vi "[FPGA] DeltaSig Main V5.vi"() -> ()   [LabVIEW 2015]
doc: "This VI provides a template for customizing a waveform acquisition using delta-sigma based NI C Series analog input smodules."
uses:
  <vilib>/LabVIEW Targets/FPGA/cRIO/shared/nicrio_ModuleControls/nicrio_cRIO-9234_ConfigModeRing.ctl
  <vilib>/rvi/Emulation/niFpgaGetClockAttributes.vi
  <vilib>/rvi/Emulation/niFpgaSctlEmulationGetInTimedLoop.vi
  <vilib>/rvi/Emulation/niFpgaEmulationReportErrorSimple.vi
  <vilib>/LabVIEW Targets/FPGA/cRIO/shared/nicrio_DsaDataRateApi/_nicrio_9234GetDataRate131.vi
  <vilib>/rvi/Emulation/niFpgaProcessEmulError.vi
  <vilib>/rvi/eio/common/nirviEmuTemplatePropertySet_errors.vi
  <vilib>/rvi/eio/common/nirviEmuTemplateMethod_errors.vi
  <vilib>/rvi/interface/RandomDataEmulation/niFpgaRandomDataHandleErrors.vi
  <vilib>/rvi/Emulation/niFpgaCriticalErrorInLSC.vi
  <vilib>/eio/EIOPropertyNode/EIOPropertyNode.xnode
  <vilib>/LabVIEW Targets/FPGA/cRIO/shared/nicrio_ModuleControls/nicrio_cRIO-9234_DataRatesRing2.ctl
  <vilib>/eio/EIONode/EIONode.xnode
  <vilib>/rvi/DataTransferAndStorage/Container/XNode/niFpgaContainer.xnode
  <vilib>/rvi/interface/RandomDataEmulation/nirviRandomDataFpgaReadWriteTemplate.vi
  <vilib>/rvi/eio/common/nirviEmuTemplatePropertyGet_errors.vi
  <vilib>/rvi/eio/common/nirviEmuTemplatePropertyGet_noerrors.vi
  <vilib>/rvi/eio/common/nirviEmuTemplatePropertySet_noerrors.vi
panel:
  in  "Array Input Config":T1[](array[typedef])=[0, 0, 0, 0, 0, 0, 0, 0, 0, 0, 0, 0, 0, 0, 0, 0, 0, 0, 0, 0, 0, 0, 0, 0] items=["AC Coupled", "DC Coupled", "IEPE AC Coupled"]
  out "oclk freq":u32
  out "oclk div":u32
  out "oclk mult":u32
  in  "data rate (S/s)":u32
  in  "Chan Scale Array":sgl[](array[numeric])=[0.0, 0.0, 0.0, 0.0, 0.0, 0.0, 0.0, 0.0, 0.0, 0.0, 0.0, 0.0, 0.0, 0.0, 0.0, 0.0, 0.0, 0.0, 0.0, 0.0, 0.0, 0.0, 0.0, 0.0, 0.0, 0.0, 0.0, 0.0, 0.0, 0.0, 0.0, 0.0, 0.0, 0.0, 0.0, 0.0, 0.0, 0.0, 0.0, 0.0]
  out "Chan Count":bool
  out "Acq Loop Ticks":u32
  out "FPGA Error":errorcluster
  out "Module Underflow":bool
  out "Finished":bool
  in  "Number of Channels":i32=24
  in  "Samps per Chan [Finite]":i32=5120
  out "First Read":bool
  in  "Acquisition Type":enum16{"Finite Samples", "Continuous Samples"}(ring)
  out "DMA FIFO Full":bool
  in  "stop":bool
  # "Array size fixed at 40\nelements but may be \nexpanded if needed"
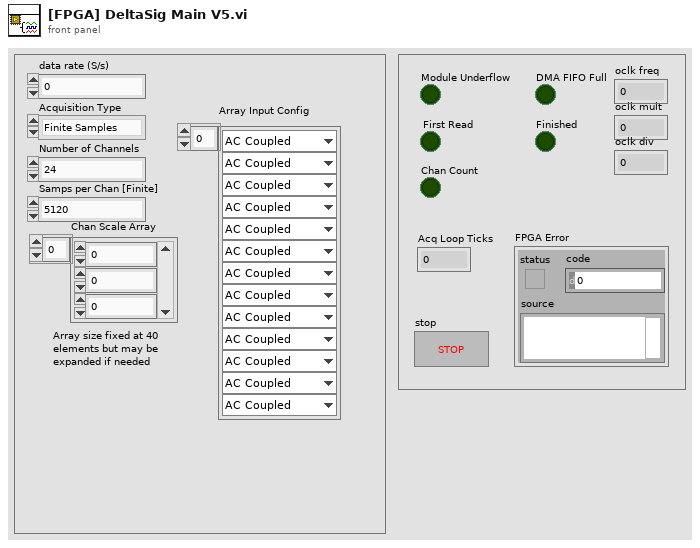
[diagram p1: front panel]
types:
  T1 = typedef "nicrio_cRIO-9234_ConfigModeRing.ctl" = u8
  T2 = typedef "nicrio_cRIO-9234_DataRatesRing2.ctl" = u8
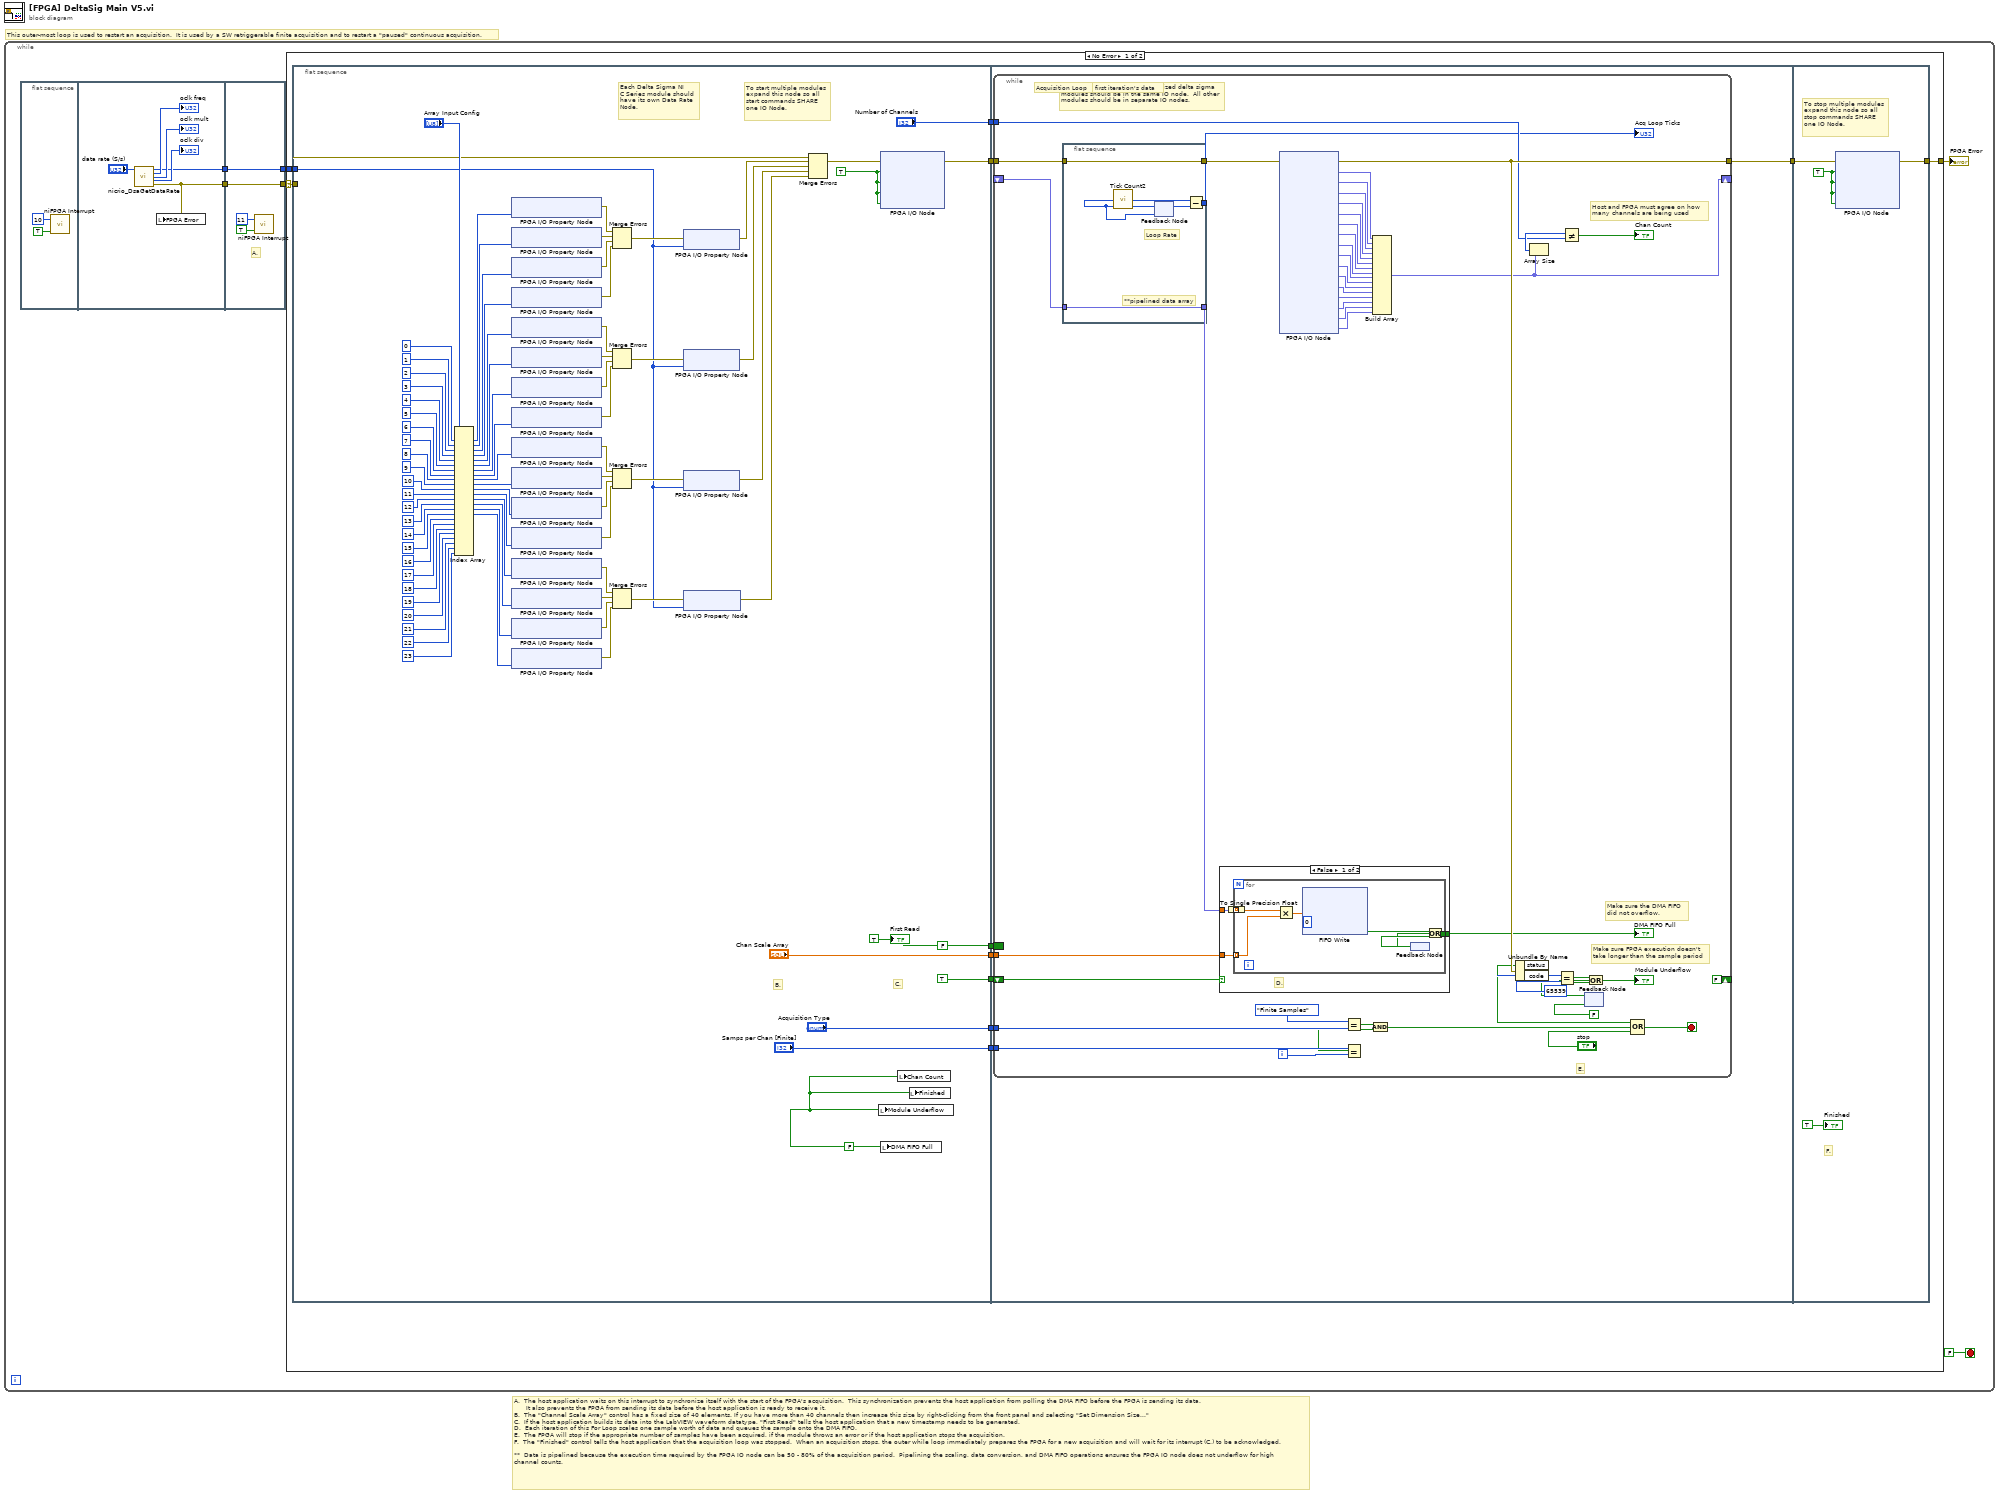
[diagram p0: block diagram]
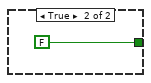
[diagram p2: hidden frame]
diagram:
  # "A.  The host application waits on this interrupt to synchronize itself with the start of the FPGA's acquisition.  This synchronization prevents the host application from polling the DMA FIFO before the FPGA is sending its data.\n      It also prevents the FPGA from sending its data before the host application is ready to receive it.\nB.  The \"Channel Scale Array\" control has a fixed size of 40 elements. If you have more than 40 channels then increase this size by right-clicking from the front panel and selecting \"Set Dimension Size...\"\nC.  If the host application builds its data into the LabVIEW waveform datatype, \"First Read\" tells the host application that a new timestamp needs to be generated.\nD.  Each iteration of this For Loop scales one sample worth of data and queues the sample onto the DMA FIFO.  \nE.  The FPGA will stop if the appropriate number of samples have been acquired, if the module throws an error or if the host application stops the acquisition.  \nF.  The \"Finished\" control tells the host application that the acquisition loop was stopped.  When an acquisition stops, the outer while loop immediately prepares the FPGA for a new acquisition and will wait for its interrupt (C.) to be acknowledged.\n\n**  Data is pipelined because the execution time required by the FPGA IO node can be 50 - 80% of the acquisition period.  Pipelining the scaling, data conversion, and DMA FIFO operations ensures the FPGA IO node does not underflow for high\nchannel counts."
  # "This outer-most loop is used to restart an acquisition.  It is used by a SW retriggerable finite acquisition and to restart a \"paused\" continuous acquisition."
  n1 = while {
    stop <- FALSE stop-if-true
    n2 = flat-sequence {
      tunnel: [w10] -> w2
      tunnel: [w11] -> w1
      tunnel: [w18] -> w3
      tunnel: [w15] -> w4
      tunnel: w2 -> [w15]
      tunnel: w1 -> [w18]
      frame #0 {
        n3 = call <vilib>:"niFPGA Interrupt.vi"("Wait Until Cleared (F)"=TRUE ("Wait Until Cleared"), "IRQ Number (0)"=u8 10 ("IRQ Number")) -> ()  [unwired: 1 in]
      }
      frame #1 {
        n4 = call-poly <vilib>:"nicrio_DsaGetDataRate.vi"("data rate (S/s)"="data rate (S/s)") -> ("data rate"=w11:T2, "oclk freq"=→"oclk freq":u32, "oclk mult"=→"oclk mult":u32, "oclk div"=→"oclk div":u32, "error out"=w10:errorcluster)  [unwired: 10 in]
        n5 = local write "FPGA Error"(w10) -> ()
      }
      frame #2 {
        # "A."
        n6 = call <vilib>:"niFPGA Interrupt.vi"("Wait Until Cleared (F)"=TRUE ("Wait Until Cleared"), "IRQ Number (0)"=u8 11 ("IRQ Number")) -> ()  [unwired: 1 in]
      }
    }
    n7 = case shown="No Error" w4 {
      selector: w4 -> [w19 w183]
      tunnel: [w21 w183] -> w5
      tunnel: w3 -> [w20 _]
      frame No Error {
        n8 = flat-sequence {
          tunnel: [w107] -> w29
          tunnel: ["Chan Scale Array"] -> w28
          tunnel: ["Acquisition Type"] -> w27
          tunnel: ["Samps per Chan [Finite]"] -> w26
          tunnel: ["Number of Channels"] -> w25
          tunnel: [TRUE ("t")] -> w24
          tunnel: [FALSE] -> w23
          tunnel: w20 -> [w30]
          tunnel: w19 -> [w79]
          tunnel: w29 -> [w114]
          tunnel: w28 -> [w113]
          tunnel: w27 -> [w111]
          tunnel: w26 -> [w110]
          tunnel: w25 -> [w115]
          tunnel: w24 -> [w112]
          tunnel: [w109] -> w22
          tunnel: w23 -> [w108]
          tunnel: w22 -> [w181]
          tunnel: [w180] -> w21
          frame #0 {
            w105 = FALSE ("Module Underflow")
            w31 = TRUE ("Mod1/Start")
            # "To start multiple modules\nexpand this node so all\nstart commands SHARE\none IO Node."
            # "C."
            # "B."
            # "Each Delta Sigma NI \nC Series module should \nhave its own Data Rate \nNode."
            n9 = Index Array(array="Array Input Config", index #1=0 ("index"), index #2=1 ("index"), index #3=2 ("index"), index #4=3 ("index"), index #5=4 ("index"), index #6=5 ("index"), index #7=6 ("index"), index #8=7 ("index"), index #9=8 ("index"), index #10=9 ("index"), index #11=10 ("index"), index #12=11 ("index"), index #13=12 ("index"), index #14=13 ("index"), index #15=14 ("index"), index #16=15 ("index"), index #17=16 ("index"), index #18=17 ("index"), index #19=18 ("index"), index #20=19 ("index"), index #21=20 ("index"), index #22=21 ("index"), index #23=22 ("index"), index #24=23 ("index")) -> (element #1=w97:T1, element #2=w96:T1, element #3=w95:T1, element #4=w94:T1, element #5=w75:T1, element #6=w74:T1, element #7=w73:T1, element #8=w72:T1, element #9=w59:T1, element #10=w58:T1, element #11=w57:T1, element #12=w56:T1, element #13=w55:T1, element #14=w53:T1, element #15=w52:T1, element #16=w51:T1)  [unwired: 8 out]
            n10 = xnode "FPGA I/O Property Node"("Input Configuration"=w97) -> ("error out"=w90:errorcluster)  [unwired: 2 in, 1 out]
            n11 = xnode "FPGA I/O Property Node"("Input Configuration"=w96) -> ("error out"=w89:errorcluster)  [unwired: 2 in, 1 out]
            n12 = xnode "FPGA I/O Property Node"("Input Configuration"=w95) -> ("error out"=w88:errorcluster)  [unwired: 2 in, 1 out]
            n13 = xnode "FPGA I/O Property Node"("Input Configuration"=w94) -> ("error out"=w87:errorcluster)  [unwired: 2 in, 1 out]
            n14 = xnode "FPGA I/O Property Node"("Input Configuration"=w75) -> ("error out"=w84:errorcluster)  [unwired: 2 in, 1 out]
            n15 = xnode "FPGA I/O Property Node"("Input Configuration"=w74) -> ("error out"=w83:errorcluster)  [unwired: 2 in, 1 out]
            n16 = xnode "FPGA I/O Property Node"("Input Configuration"=w73) -> ("error out"=w82:errorcluster)  [unwired: 2 in, 1 out]
            n17 = xnode "FPGA I/O Property Node"("Input Configuration"=w72) -> ("error out"=w81:errorcluster)  [unwired: 2 in, 1 out]
            n18 = xnode "FPGA I/O Property Node"("Input Configuration"=w59) -> ("error out"=w67:errorcluster)  [unwired: 2 in, 1 out]
            n19 = xnode "FPGA I/O Property Node"("Input Configuration"=w58) -> ("error out"=w66:errorcluster)  [unwired: 2 in, 1 out]
            n20 = xnode "FPGA I/O Property Node"("Input Configuration"=w57) -> ("error out"=w65:errorcluster)  [unwired: 2 in, 1 out]
            n21 = xnode "FPGA I/O Property Node"("Input Configuration"=w56) -> ("error out"=w64:errorcluster)  [unwired: 2 in, 1 out]
            n22 = xnode "FPGA I/O Property Node"("Input Configuration"=w55) -> ("error out"=w63:errorcluster)  [unwired: 2 in, 1 out]
            n23 = xnode "FPGA I/O Property Node"("Input Configuration"=w53) -> ("error out"=w62:errorcluster)  [unwired: 2 in, 1 out]
            n24 = xnode "FPGA I/O Property Node"("Input Configuration"=w52) -> ("error out"=w61:errorcluster)  [unwired: 2 in, 1 out]
            n25 = xnode "FPGA I/O Property Node"("Input Configuration"=w51) -> ("error out"=w60:errorcluster)  [unwired: 2 in, 1 out]
            n26 = Merge Errors(w90, w89, w88, w87) -> (w86:errorcluster)
            n27 = Merge Errors(w84, w83, w82, w81) -> (w80:errorcluster)
            n28 = Merge Errors(w67, w66, w65, w64) -> (w54:errorcluster)
            n29 = Merge Errors(w63, w62, w61, w60) -> (w34:errorcluster)
            n30 = xnode "FPGA I/O Property Node"("error in"=w86, "Data Rate"=w30) -> ("error out"=w77:errorcluster)  [unwired: 1 in, 1 out]
            n31 = xnode "FPGA I/O Property Node"("error in"=w80, "Data Rate"=w30) -> ("error out"=w76:errorcluster)  [unwired: 1 in, 1 out]
            n32 = xnode "FPGA I/O Property Node"("error in"=w54, "Data Rate"=w30) -> ("error out"=w33:errorcluster)  [unwired: 1 in, 1 out]
            n33 = xnode "FPGA I/O Property Node"("error in"=w34, "Data Rate"=w30) -> ("error out"=w32:errorcluster)  [unwired: 1 in, 1 out]
            n34 = Merge Errors(w79, w77, w76, w33, w32) -> (w78:errorcluster)
            n35 = local write "Module Underflow"(w105) -> ()
            n36 = xnode "FPGA I/O Node"("error in"=w78, "Mod1/Start"=w31, "Mod2/Start"=w31, "Mod3/Start"=w31, "Mod4/Start"=w31) -> ("error out"=w107:errorcluster)  [unwired: 4 in, 4 out]
            n37 = local write "DMA FIFO Full"(w105) -> ()
            n38 = local write "Chan Count"(w105) -> ()
            n39 = local write "Finished"(w105) -> ()
            "First Read" <- TRUE ("First Read")
          }
          frame #1 {
            n40 = while {
              tunnel: w114 -> [w151]
              tunnel: [w156] -> w109
              tunnel: w111 -> [w158]
              tunnel: w110 -> [w157]
              shift-right: [w131] -> _
              shift-left: _ -> [w144]
              tunnel: w115 -> [w153]
              tunnel: w113 -> [w145]
              shift-right: [FALSE ("t")] -> _
              shift-left: w112 -> [w143]
              border: w108 -> [_]
              i -> [w141]
              stop <- w128 stop-if-true
              # "Add channels here.  All synchronized delta sigma\nmodules should be in the same IO node.  All other\nmodules should be in separate IO nodes."
              # "Do not DMA first iteration's data"
              # "Acquisition Loop"
              # "E."
              # "Host and FPGA must agree on how \nmany channels are being used"
              # "Make sure the DMA FIFO\ndid not overflow."
              # "Make sure FPGA execution doesn't\ntake longer than the sample period"
              n41 = flat-sequence {
                tunnel: [w178] -> w150
                tunnel: w151 -> [w178]
                tunnel: [w175] -> w149
                tunnel: w144 -> [w174]
                tunnel: [w174] -> w130
                frame #0 {
                  # "**pipelined data array"
                  # "Loop Rate"
                  n42 = call "Tick Count2"() -> ("Tick Count(Ticks)"=w177:u32)
                  n43 = feedback-in #1(w177) -> ()
                  n44 = feedback #1(w177) -> (w176:u32)
                  n45 = Subtract(x=w177, y=w176) -> (x-y=w175:u32)
                }
              }
              n46 = To Single Precision Float(number=w130) -> (single precision float=w129:sgl[])
              n47 = case shown="False" w143 {
                tunnel: [w165 FALSE] -> w155
                tunnel: w145 -> [w164 _]
                tunnel: w129 -> [w163 _]
                frame False {
                  # "D."
                  n48 = for {
                    tunnel: [w170] -> w165
                    tunnel: w163 -> [w168] mode=indexing
                    tunnel: w164 -> [w167] mode=indexing
                    n49 = Multiply(x=w168, y=w167) -> (x*y=w166:sgl)
                    n50 = xnode ("FIFO Write")("Element"=w166, "Timeout"=0) -> ("Timed Out?"=w172:bool)  [unwired: 1 in, 1 out]
                    n51 = feedback #2() -> (w171:bool)
                    n52 = Or(x=w172, y=w171) -> (x .or. y?=w170:bool)
                    n53 = feedback-in #2(w170) -> ()
                  }
                }
                frame True {
                }
              }
              "DMA FIFO Full" <- w155
              n54 = xnode "FPGA I/O Node"("error in"=w150) -> ("error out"=w156:errorcluster, "Mod1/AI0"=w148:fxp<+/-,24,4>, "Mod1/AI1"=w140:fxp<+/-,24,4>, "Mod1/AI2"=w147:fxp<+/-,24,4>, "Mod1/AI3"=w146:fxp<+/-,24,4>, "Mod2/AI0"=w127:fxp<+/-,24,4>, "Mod2/AI1"=w126:fxp<+/-,24,4>, "Mod2/AI2"=w125:fxp<+/-,24,4>, "Mod2/AI3"=w124:fxp<+/-,24,4>, "Mod3/AI0"=w123:fxp<+/-,24,4>, "Mod3/AI1"=w122:fxp<+/-,24,4>, "Mod3/AI2"=w121:fxp<+/-,24,4>, "Mod3/AI3"=w120:fxp<+/-,24,4>, "Mod4/AI0"=w119:fxp<+/-,24,4>, "Mod4/AI1"=w118:fxp<+/-,24,4>, "Mod4/AI2"=w117:fxp<+/-,24,4>, "Mod4/AI3"=w116:fxp<+/-,24,4>)  [unwired: 16 in, 16 out]
              n55 = Equal?(x=enum16{"Finite Samples", "Continuous Samples"}."Finite Samples" ("y"), y=w158) -> (x = y?=w134:bool)
              n56 = Equal?(x=w157, y=w141) -> (x = y?=w133:bool)
              n57 = And(x=w134, y=w133) -> (x .and. y?=w132:bool)
              n58 = Build Array(w148, w140, w147, w146, w127, w126, w125, w124, w123, w122, w121, w120, w119, w118, w117, w116) -> (w131:fxp<+/-,24,4>[])
              n59 = Unbundle By Name(w156) -> ("status"=w139:bool, "code"=w159:i32)
              n60 = Array Size(array=w131) -> (size(s)=w154:i32)
              n61 = Equal?(x=w159, y=65539) -> (x = y?=w136:bool)
              n62 = Not Equal?(x=w154, y=w153) -> (x != y?=→"Chan Count":bool)
              n63 = feedback #3(FALSE) -> (w138:bool)
              n64 = Or(x=w136, y=w138) -> (x .or. y?=w135:bool)
              "Module Underflow" <- w135
              n65 = feedback-in #3(w135) -> ()
              n66 = Compound Arithmetic op=OR(w139, w132, "stop") -> (w128:bool)
              "Acq Loop Ticks" <- w149
            }
          }
          frame #2 {
            w179 = TRUE ("Mod1/Stop")
            # "To stop multiple modules\nexpand this node so all\nstop commands SHARE\none IO Node."
            # "F."
            n67 = xnode "FPGA I/O Node"("error in"=w181, "Mod1/Stop"=w179, "Mod2/Stop"=w179, "Mod3/Stop"=w179, "Mod4/Stop"=w179) -> ("error out"=w180:errorcluster)  [unwired: 4 in, 4 out]
            "Finished" <- TRUE ("Finished")
          }
        }
      }
      frame Error {
      }
    }
    "FPGA Error" <- w5
  }
